vi "Project Spec Type.vi"(0 "NI Build Specification in":refnum<class "NIPKG_LV.lvclass">, 11 "error in (no error)":errorcluster) -> (4 "NI Build Specification out":refnum<class "NIPKG_LV.lvclass">, 6 "Project Specfication Type":string, 15 "error out":errorcluster)   [LabVIEW 2017, in "CL_G3_VIComponentBuilder.lvlib" / "NIPKG_LV.lvclass"]
doc: "Returns the GUID as defined by NI used for NI Package build spec type."
uses:
  NIPKG_LV.lvclass
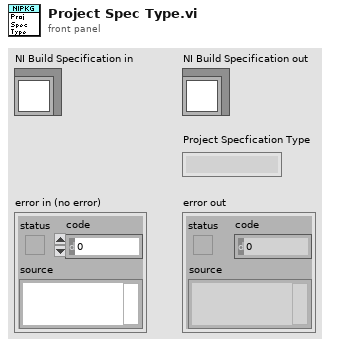
[diagram p1: front panel]
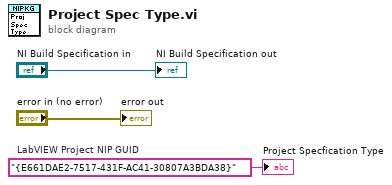
[diagram p0: block diagram]
diagram:
  w1 = "{E661DAE2-7517-431F-AC41-30807A3BDA38}"  # LabVIEW Project NIP GUID
  "error out" <- "error in (no error)"
  "NI Build Specification out" <- "NI Build Specification in"
  "Project Specfication Type" <- w1
